vi "test.vi"() -> ()   [LabVIEW 2016, in "labssh_thijs.lvlib"]
uses:
  labssh_thijs.lvlib
  state machine.ctl
panel:
  out "error out":errorcluster
  out "output":string
  in  "input":string
  in  "New Button":bool
  in  "OK Button":bool
  in  "Stop Button":bool
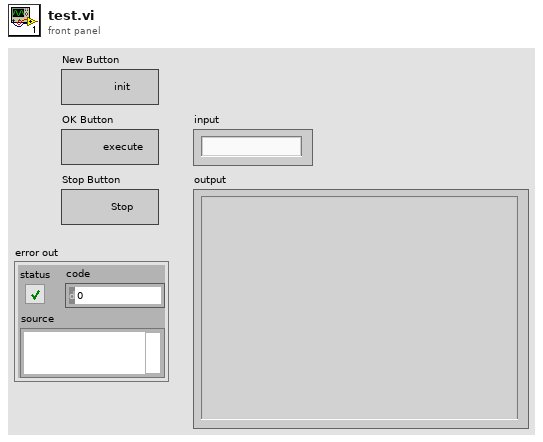
[diagram p1: front panel]
types:
  T1 = typedef "labssh_thijs.lvlib/state machine.ctl" = enum16{"init", "connect", "execute", "close", "exit", "read"}
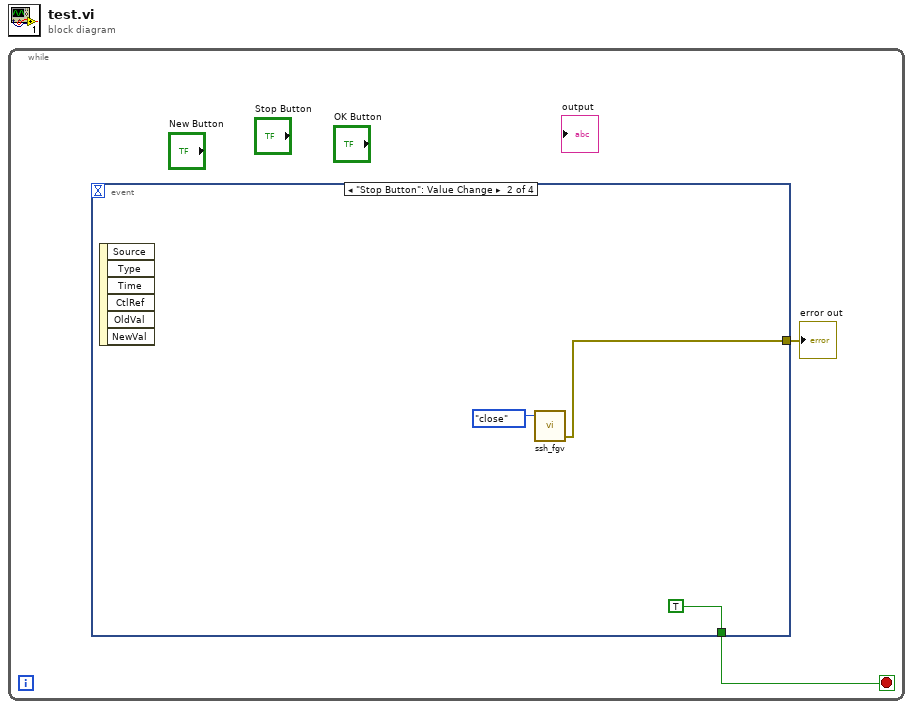
[diagram p0: block diagram]
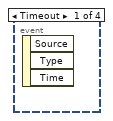
[diagram p2: hidden frame]
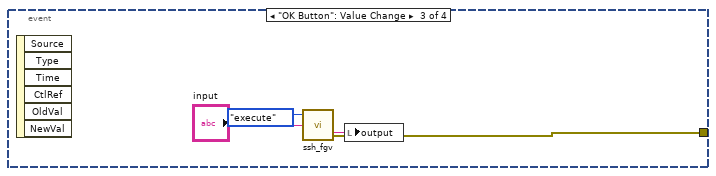
[diagram p3: hidden frame]
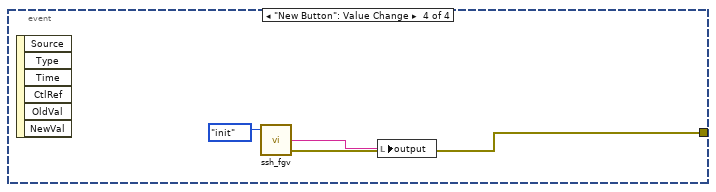
[diagram p4: hidden frame]
diagram:
  n1 = while {
    stop <- w2 stop-if-true
    n2 = event shown="[1] \"Stop Button\": Value Change" {
      selector: _ -> [_ _ _ _]
      dyn-events: _ -> [_ _ _ _]
      timeout: _ -> [_ _ _ _]
      tunnel: [_ TRUE _ _] -> w2
      tunnel: [_ w4 w7 w10] -> w1
      event Timeout {
        n3 = event-data() -> ()  [unwired: 1 in, 3 out]
      }
      event "Stop Button": Value Change {
        n4 = event-data() -> ()  [unwired: 1 in, 6 out]
        n5 = call "ssh_fgv.vi"("state"=state_machine."close") -> ("error out"=w4:errorcluster)  [unwired: 3 in, 1 out]
      }
      event "OK Button": Value Change {
        n6 = event-data() -> ()  [unwired: 1 in, 6 out]
        n7 = call "ssh_fgv.vi"("Input"="input", "state"=state_machine."execute") -> ("error out"=w7:errorcluster, "output_new"=w8:string)  [unwired: 2 in]
        n8 = local write "output"(w8) -> ()
      }
      event "New Button": Value Change {
        n9 = event-data() -> ()  [unwired: 1 in, 6 out]
        n10 = call "ssh_fgv.vi"("state"=state_machine."init") -> ("error out"=w10:errorcluster, "output_new"=w11:string)  [unwired: 3 in]
        n11 = local write "output"(w11) -> ()
      }
    }
    "error out" <- w1
  }
